vi "Part 1.vi"(11 "Input":string) -> (3 "Output":i32)   [LabVIEW 2021]
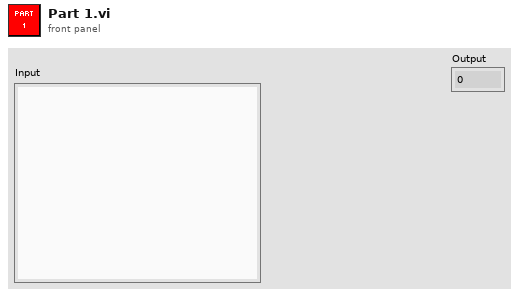
[diagram p1: front panel]
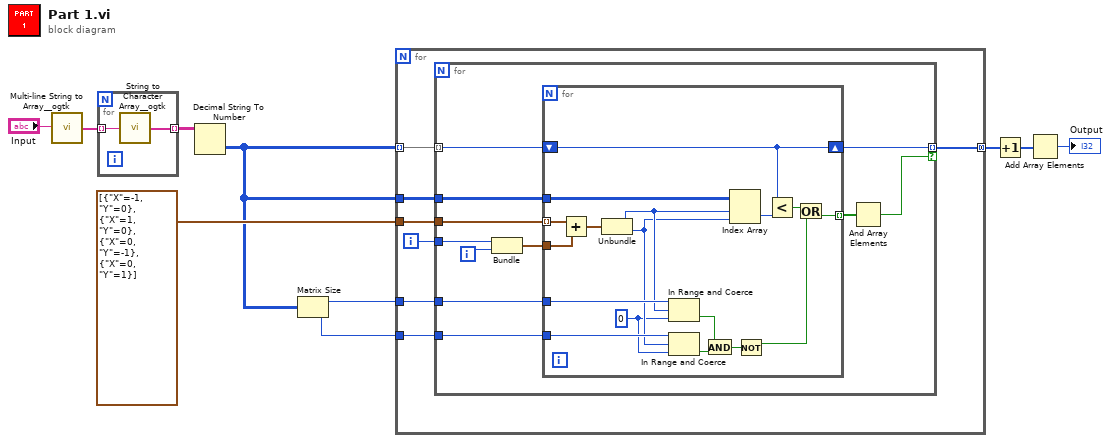
[diagram p0: block diagram]
diagram:
  n1 = call <userlib>:"Multi-line String to Array__ogtk.vi"("string"="Input") -> ("lines"=w9:string[])
  n2 = for {
    tunnel: w9 -> [w12] mode=indexing
    tunnel: [w11] -> w8 mode=indexing
    n3 = call <userlib>:"String to Character Array__ogtk.vi"("Input String"=w12) -> ("Character Array"=w11:string[])
  }
  n4 = Decimal String To Number(string=w8) -> (number=w3:i32[][])  [unwired: 2 in, 1 out]
  n5 = Matrix Size(0:w3) -> (1:w2:i32, 2:w1:i32)
  n6 = for {
    tunnel: w3 -> [w19] mode=indexing
    tunnel: w3 -> [w18]
    tunnel: cluster{"X":i32, "Y":i32}[] [{"X"=-1, "Y"=0}, {"X"=1, "Y"=0}, {"X"=0, "Y"=-1}, {"X"=0, "Y"=1}] -> [w17]
    tunnel: [w15] -> w6 mode=concatenating
    tunnel: w2 -> [w14]
    tunnel: w1 -> [w13]
    i -> [w16]
    n7 = for {
      tunnel: w19 -> [w28] mode=indexing
      tunnel: w18 -> [w30]
      tunnel: w17 -> [w29]
      tunnel: w16 -> [w27]
      tunnel: [w23] -> w15 mode=indexing if=w22
      tunnel: w14 -> [w21]
      tunnel: w13 -> [w20]
      i -> [w26]
      n8 = Bundle(w27, w26) -> (w25:cluster{i32, i32})  [unwired: 1 in]
      n9 = for {
        tunnel: w30 -> [w47]
        tunnel: w29 -> [w46] mode=indexing
        tunnel: w25 -> [w45]
        tunnel: [w32] -> w24 mode=indexing
        shift-right: [w41] -> w23
        shift-left: w28 -> [w41]
        tunnel: w21 -> [w40]
        tunnel: w20 -> [w38]
        w36 = 0 ("lower limit")
        n10 = Add(x=w46, y=w45) -> (x+y=w44:cluster{i32, i32})
        n11 = Unbundle(w44) -> (w39:i32, w37:i32)
        n12 = In Range and Coerce(upper limit=w40, x=w39, lower limit=w36) -> (In Range?=w34:bool)  [unwired: 1 out]
        n13 = In Range and Coerce(upper limit=w38, x=w37, lower limit=w36) -> (In Range?=w35:bool)  [unwired: 1 out]
        n14 = And(x=w34, y=w35) -> (x .and. y?=w33:bool)
        n15 = Index Array(array=w47, index (row)=w39, index (col)=w37) -> (element=w43:i32)
        n16 = Not(x=w33) -> (.not. x?=w31:bool)
        n17 = Less?(x=w41, y=w43) -> (x < y?=w42:bool)
        n18 = Or(x=w42, y=w31) -> (x .or. y?=w32:bool)
      }
      n19 = And Array Elements(Boolean array=w24) -> (logical AND=w22:bool)
    }
  }
  n20 = Increment(x=w6) -> (x+1=w5:i32[])
  n21 = Add Array Elements(numeric array=w5) -> (sum=→"Output":i32)
